vi "CAN总线测试.vi"() -> ()   [LabVIEW 2010]
uses:
  全局量/试验配置信息.vi
panel:
  in  "同步_2":i32
  in  "同步_1":i32
  out "CAN_R_4_4":u16
  out "CAN_R_4_3":u16
  out "CAN_R_4_2":u16
  out "CAN_R_4_1":u16
  out "CAN_R_3_4":u16
  out "CAN_R_3_3":u16
  out "CAN_R_3_2":u16
  out "CAN_R_3_1":u16
  out "CAN_R_2_4":u16
  out "CAN_R_2_3":u16
  out "CAN_R_2_2":u16
  out "CAN_R_2_1":u16
  out "CAN_R_1_4":u16
  out "CAN_R_1_3":u16
  out "CAN_R_1_2":u16
  out "CAN_R_1_1":u16
  out "结束?":bool
  out "light_4":bool
  out "light_3":bool
  out "light_2":bool
  out "light_1":bool
  out "测试结论":string
  in  "btn_关闭":bool
  in  "btn_开始测试":bool
  in  "CAN_4_4":u16
  in  "CAN_4_3":u16
  in  "CAN_4_2":u16
  in  "CAN_4_1":u16
  in  "单选_CAN_4":bool
  in  "CAN_3_4":u16
  in  "CAN_3_3":u16
  in  "CAN_3_2":u16
  in  "CAN_3_1":u16
  in  "单选_CAN_3":bool
  in  "CAN_2_4":u16
  in  "CAN_2_3":u16
  in  "CAN_2_2":u16
  in  "CAN_2_1":u16
  in  "单选_CAN_2":bool
  in  "CAN_1_4":u16
  in  "CAN_1_3":u16
  in  "CAN_1_2":u16
  in  "CAN_1_1":u16
  in  "单选_CAN_1":bool
  # "CAN以发送数据："
  # "CAN1"
  # "CAN2"
  # "CAN3"
  # "CAN4"
  # "CAN接收数据："
  # "CAN1"
  # "CAN2"
  # "CAN3"
  # "CAN4"
  # "测试结论："
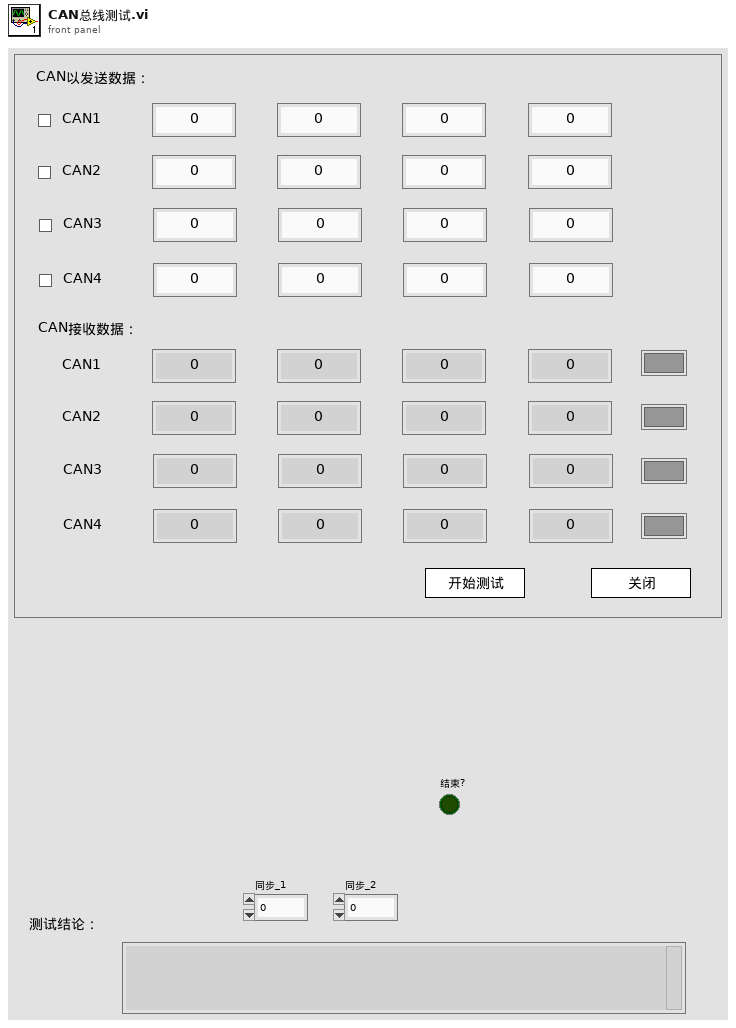
[diagram p1: front panel]
types:
  T1 = enum8{"Enabled", "Disabled", "Disabled and Grayed Out"}
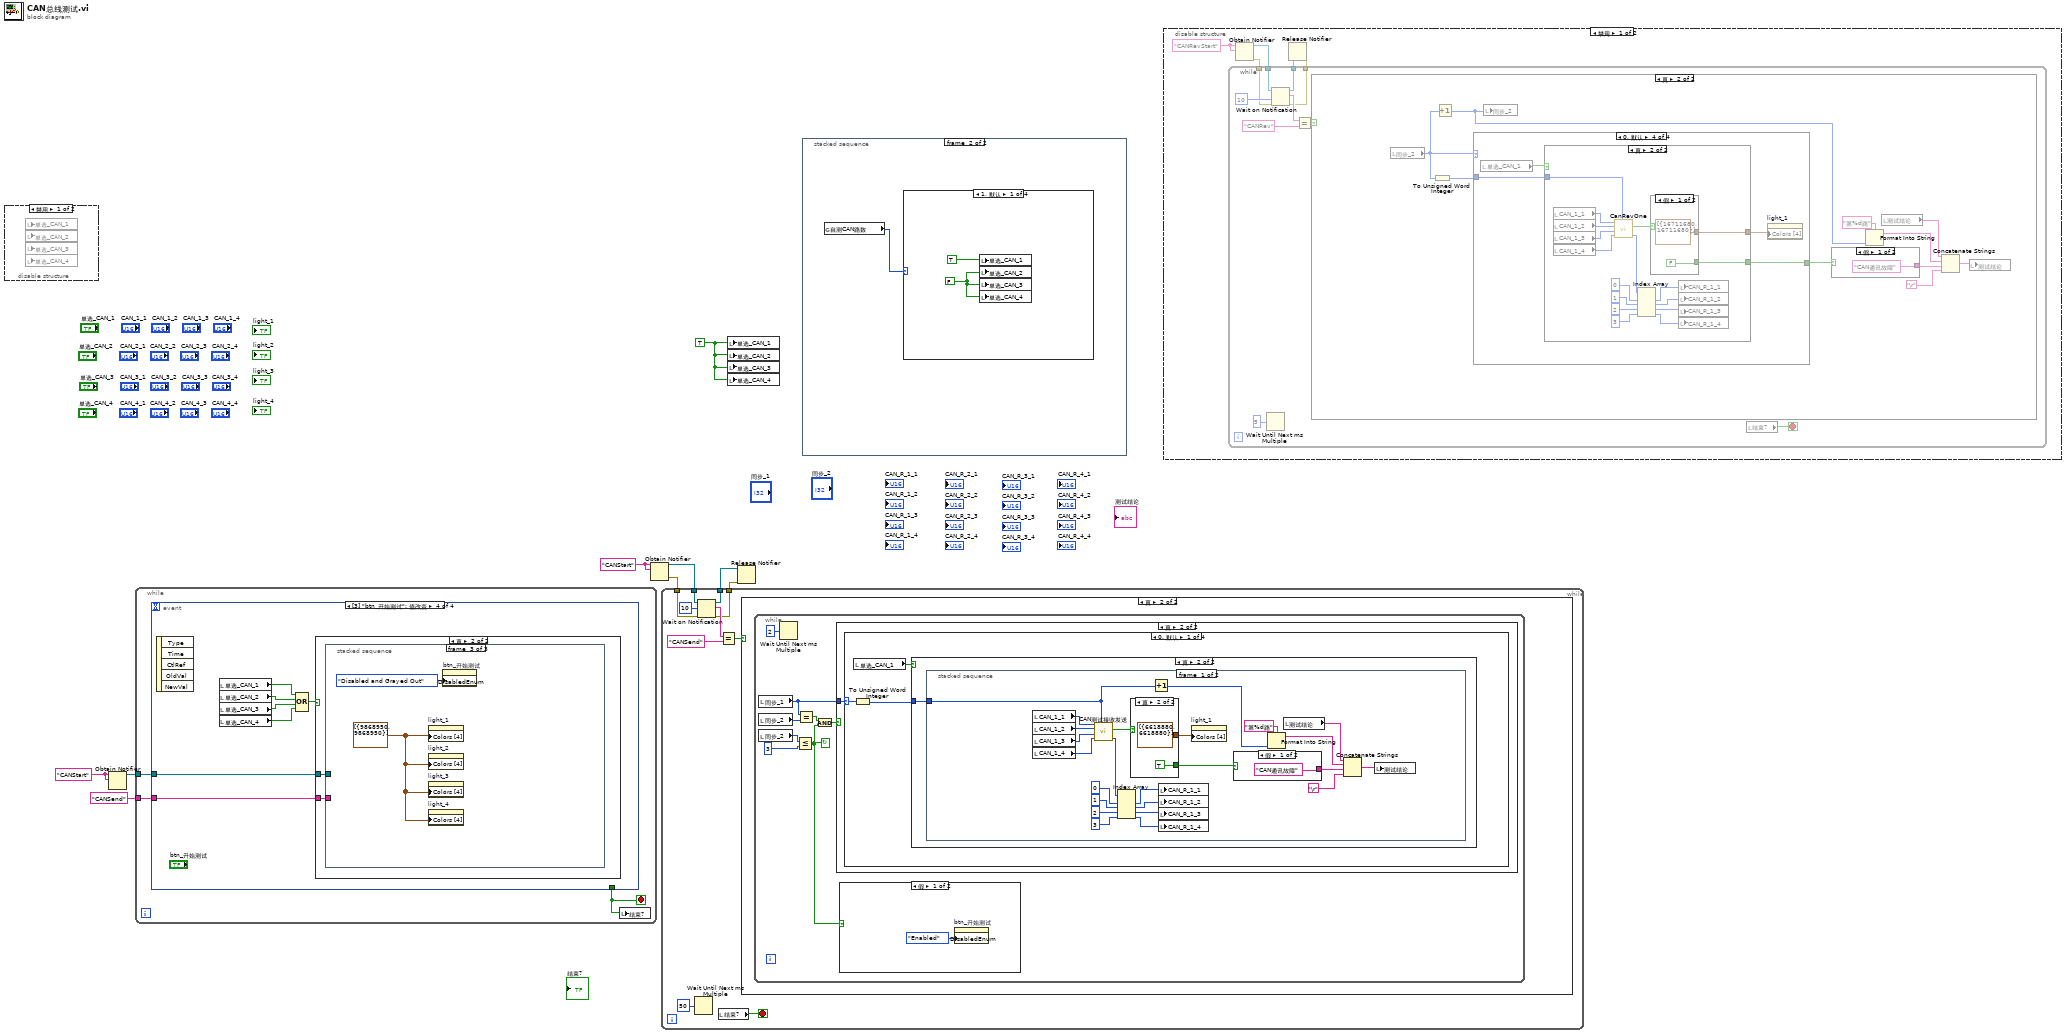
[diagram p0: block diagram]
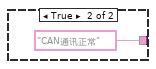
[diagram p3: hidden frame]
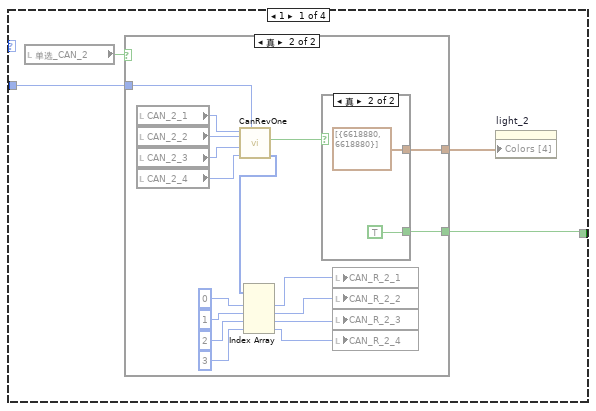
[diagram p4: hidden frame]
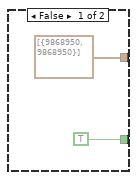
[diagram p5: hidden frame]
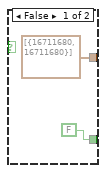
[diagram p6: hidden frame]
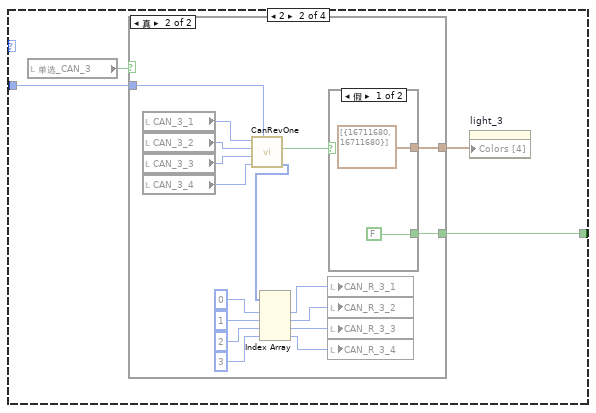
[diagram p7: hidden frame]
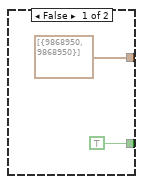
[diagram p8: hidden frame]
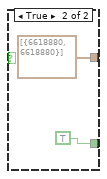
[diagram p9: hidden frame]
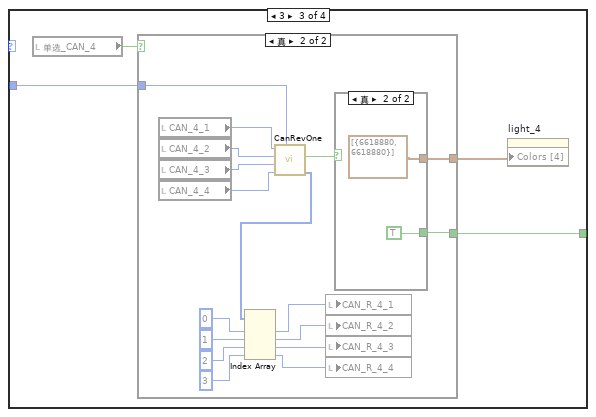
[diagram p10: hidden frame]
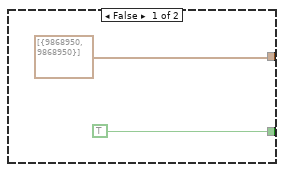
[diagram p11: hidden frame]
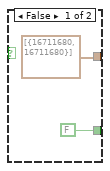
[diagram p12: hidden frame]
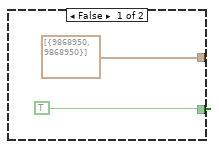
[diagram p13: hidden frame]
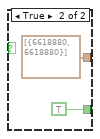
[diagram p14: hidden frame]
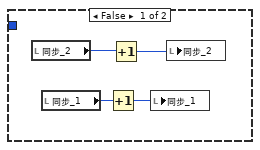
[diagram p19: hidden frame]
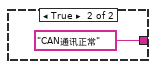
[diagram p20: hidden frame]
diagram:
  w1 = TRUE ("单选_CAN_1")
  w4 = "CANStart" ("名称（未命名）")
  w9 = "CANStart" ("名称（未命名）")
  n1 = disable-structure shown="禁用" {
    frame Disabled {
      n2 = local read "单选_CAN_1"() -> ()  [unwired: 1 in]
      n3 = local read "单选_CAN_2"() -> ()  [unwired: 1 in]
      n4 = local read "单选_CAN_3"() -> ()  [unwired: 1 in]
      n5 = local read "单选_CAN_4"() -> ()  [unwired: 1 in]
    }
    frame Enabled {
    }
  }
  n6 = Obtain Notifier(name (unnamed)=w4, notification data type=w4) -> (notifier out=w3:refnum<notifier>)  [unwired: 2 in, 2 out]
  n7 = while {
    tunnel: w3 -> [w11]
    tunnel: "CANSend" ("通知") -> [w10]
    stop <- w12 stop-if-true
    n8 = event shown="[3] \"btn_开始测试\": 值改变" {
      selector: _ -> [_ _ _ _]
      dyn-events: _ -> [_ _ _ _]
      timeout: _ -> [_ _ _ _]
      tunnel: [_ TRUE TRUE _] -> w12
      tunnel: w11 -> [_ _ _ w22]
      tunnel: w10 -> [_ _ _ w21]
      event Timeout {
        n9 = event-data() -> ()  [unwired: 1 in, 2 out]
      }
      event Panel Close {
        n10 = event-data() -> ()  [unwired: 1 in, 3 out]
        n11 = stacked-sequence {
          frame #0 {
            w14 = u16 0 ("CAN_R_1_1")
            w15 = 0 ("同步_2")
            w16 = cluster{u32, u32}[] [{9868950, 9868950}]
            n12 = local write "同步_2"(w15) -> ()
            n13 = local write "同步_1"(w15) -> ()
            n14 = property on="light_1" class="Bool (严格)"("Colors [4]"=w16) -> ()  [unwired: 2 in, 2 out]
            n15 = property on="light_2" class="Bool (严格)"("Colors [4]"=w16) -> ()  [unwired: 2 in, 2 out]
            n16 = property on="light_3" class="Bool (严格)"("Colors [4]"=w16) -> ()  [unwired: 2 in, 2 out]
            n17 = property on="light_4" class="Bool (严格)"("Colors [4]"=w16) -> ()  [unwired: 2 in, 2 out]
            n18 = local write "CAN_R_1_1"(w14) -> ()
            n19 = local write "CAN_R_1_2"(w14) -> ()
            n20 = local write "CAN_R_1_3"(w14) -> ()
            n21 = local write "CAN_R_1_4"(w14) -> ()
            n22 = local write "CAN_R_2_1"(w14) -> ()
            n23 = local write "CAN_R_2_2"(w14) -> ()
            n24 = local write "CAN_R_2_3"(w14) -> ()
            n25 = local write "CAN_R_2_4"(w14) -> ()
            n26 = local write "CAN_R_3_1"(w14) -> ()
            n27 = local write "CAN_R_3_2"(w14) -> ()
            n28 = local write "CAN_R_3_3"(w14) -> ()
            n29 = local write "CAN_R_3_4"(w14) -> ()
            n30 = local write "CAN_R_4_1"(w14) -> ()
            n31 = local write "CAN_R_4_2"(w14) -> ()
            n32 = local write "CAN_R_4_3"(w14) -> ()
            n33 = local write "CAN_R_4_4"(w14) -> ()
          }
        }
      }
      event "btn_关闭": Value Change {
        n34 = event-data() -> ()  [unwired: 1 in, 5 out]
        n35 = stacked-sequence {
          frame #0 {
            w18 = u16 0 ("CAN_R_1_1")
            w19 = 0 ("同步_2")
            w20 = cluster{u32, u32}[] [{9868950, 9868950}]
            n36 = local write "同步_2"(w19) -> ()
            n37 = local write "同步_1"(w19) -> ()
            n38 = property on="light_1" class="Bool (严格)"("Colors [4]"=w20) -> ()  [unwired: 2 in, 2 out]
            n39 = property on="light_2" class="Bool (严格)"("Colors [4]"=w20) -> ()  [unwired: 2 in, 2 out]
            n40 = property on="light_3" class="Bool (严格)"("Colors [4]"=w20) -> ()  [unwired: 2 in, 2 out]
            n41 = property on="light_4" class="Bool (严格)"("Colors [4]"=w20) -> ()  [unwired: 2 in, 2 out]
            n42 = local write "CAN_R_1_1"(w18) -> ()
            n43 = local write "CAN_R_1_2"(w18) -> ()
            n44 = local write "CAN_R_1_3"(w18) -> ()
            n45 = local write "CAN_R_1_4"(w18) -> ()
            n46 = local write "CAN_R_2_1"(w18) -> ()
            n47 = local write "CAN_R_2_2"(w18) -> ()
            n48 = local write "CAN_R_2_3"(w18) -> ()
            n49 = local write "CAN_R_2_4"(w18) -> ()
            n50 = local write "CAN_R_3_1"(w18) -> ()
            n51 = local write "CAN_R_3_2"(w18) -> ()
            n52 = local write "CAN_R_3_3"(w18) -> ()
            n53 = local write "CAN_R_3_4"(w18) -> ()
            n54 = local write "CAN_R_4_1"(w18) -> ()
            n55 = local write "CAN_R_4_2"(w18) -> ()
            n56 = local write "CAN_R_4_3"(w18) -> ()
            n57 = local write "CAN_R_4_4"(w18) -> ()
          }
        }
      }
      event "btn_开始测试": Value Change {
        n58 = event-data() -> ()  [unwired: 1 in, 5 out]
        n59 = local read "单选_CAN_1"() -> (w27:bool)
        n60 = local read "单选_CAN_2"() -> (w26:bool)
        n61 = local read "单选_CAN_3"() -> (w25:bool)
        n62 = local read "单选_CAN_4"() -> (w24:bool)
        n63 = Compound Arithmetic op=OR(w27, w26, w25, w24) -> (w23:bool)
        n64 = case shown="真" w23 {
          tunnel: w22 -> [_ w29]
          tunnel: w21 -> [_ w28]
          frame False {
            n65 = call "显示对话框信息"() -> ()  [unwired: 10 in, 2 out]
          }
          frame True {
            n66 = stacked-sequence {
              tunnel: w29 -> [_ w34 _]
              tunnel: w28 -> [_ w33 _]
              frame #0 {
                w30 = u16 0 ("CAN_R_1_1")
                w31 = 0 ("同步_2")
                n67 = local write "同步_2"(w31) -> ()
                n68 = local write "同步_1"(w31) -> ()
                n69 = local write "测试结论"("") -> ()
                n70 = local write "CAN_R_1_1"(w30) -> ()
                n71 = local write "CAN_R_1_2"(w30) -> ()
                n72 = local write "CAN_R_1_3"(w30) -> ()
                n73 = local write "CAN_R_1_4"(w30) -> ()
                n74 = local write "CAN_R_2_1"(w30) -> ()
                n75 = local write "CAN_R_2_2"(w30) -> ()
                n76 = local write "CAN_R_2_3"(w30) -> ()
                n77 = local write "CAN_R_2_4"(w30) -> ()
                n78 = local write "CAN_R_3_1"(w30) -> ()
                n79 = local write "CAN_R_3_2"(w30) -> ()
                n80 = local write "CAN_R_3_3"(w30) -> ()
                n81 = local write "CAN_R_3_4"(w30) -> ()
                n82 = local write "CAN_R_4_1"(w30) -> ()
                n83 = local write "CAN_R_4_2"(w30) -> ()
                n84 = local write "CAN_R_4_3"(w30) -> ()
                n85 = local write "CAN_R_4_4"(w30) -> ()
              }
              frame #1 {
                n86 = Send Notification(notification=w33, notifier=w34) -> ()  [unwired: 1 in, 2 out]
              }
              frame #2 {
                w35 = cluster{u32, u32}[] [{9868950, 9868950}]
                n87 = property on="light_1" class="Bool (严格)"("Colors [4]"=w35) -> ()  [unwired: 2 in, 2 out]
                n88 = property on="light_2" class="Bool (严格)"("Colors [4]"=w35) -> ()  [unwired: 2 in, 2 out]
                n89 = property on="light_3" class="Bool (严格)"("Colors [4]"=w35) -> ()  [unwired: 2 in, 2 out]
                n90 = property on="light_4" class="Bool (严格)"("Colors [4]"=w35) -> ()  [unwired: 2 in, 2 out]
                n91 = property on="btn_开始测试" class="Bool"("DisabledEnum"=T1."Disabled and Grayed Out" ("禁用")) -> ()  [unwired: 2 in, 2 out]
              }
            }
          }
        }
      }
    }
    n92 = local write "结束?"(w12) -> ()
  }
  n93 = Obtain Notifier(name (unnamed)=w9, notification data type=w9) -> (notifier out=w7:refnum<notifier>, error out=w8:errorcluster)  [unwired: 2 in, 1 out]
  n94 = while {
    tunnel: w8 -> [w40]
    tunnel: w7 -> [w39]
    tunnel: [w38] -> w6
    tunnel: [w37] -> w5
    stop <- w45 stop-if-true
    n95 = Wait Until Next ms Multiple(millisecond multiple=u32 50 ("毫秒倍数")) -> ()  [unwired: 1 out]
    n96 = Wait on Notification(notifier=w39, timeout in ms (-1)=10 ("超时毫秒(-1)"), error in (no error)=w40) -> (notifier out=w38:refnum<notifier>, notification=w42:string, error out=w37:errorcluster)  [unwired: 1 in, 1 out]
    n97 = local read "结束?"() -> (w45:bool)
    n98 = Equal?(x=w42, y="CANSend" ("通知")) -> (x = y?=w41:bool)
    n99 = case shown="真" w41 {
      frame False {
      }
      frame True {
        n100 = while {
          stop <- w47 continue-if-true
          n101 = local read "同步_1"() -> (w54:i32)
          n102 = local read "同步_2"() -> (w50:i32)
          n103 = local read "同步_2"() -> (w52:i32)
          n104 = Wait Until Next ms Multiple(millisecond multiple=u32 2 ("毫秒倍数")) -> ()  [unwired: 1 out]
          n105 = Less Or Equal?(x=w52, y=3) -> (x <= y?=w47:bool)
          n106 = Equal?(x=w54, y=w50) -> (x = y?=w48:bool)
          n107 = And(x=w48, y=w47) -> (x .and. y?=w49:bool)
          n108 = case shown="真" w49 {
            tunnel: w54 -> [_ w56]
            frame False {
            }
            frame True {
              n109 = case shown="0, 默认" w56 {
                selector: w56 -> [w57 w101 w143 w185]
                frame 0, Default {
                  n110 = local read "单选_CAN_1"() -> (w59:bool)
                  n111 = To Unsigned Word Integer(number=w57) -> (unsigned 16bit integer=w58:u16)
                  n112 = case shown="真" w59 {
                    tunnel: w58 -> [_ w64]
                    frame False {
                      n113 = local read "同步_2"() -> (w62:i32)
                      n114 = local read "同步_1"() -> (w60:i32)
                      n115 = Increment(x=w60) -> (x+1=w61:i32)
                      n116 = Increment(x=w62) -> (x+1=w63:i32)
                      n117 = local write "同步_1"(w61) -> ()
                      n118 = local write "同步_2"(w63) -> ()
                    }
                    frame True {
                      n119 = stacked-sequence {
                        tunnel: w64 -> [w65 _]
                        frame #0 {
                          n120 = local read "CAN_1_1"() -> (w75:u16)
                          n121 = local read "CAN_1_2"() -> (w76:u16)
                          n122 = local read "CAN_1_3"() -> (w77:u16)
                          n123 = local read "CAN_1_4"() -> (w78:u16)
                          n124 = call "CAN测试接收发送.vi"("Order"=w65, "data_4"=w78, "data_3"=w77, "data_2"=w76, "data_1"=w75) -> ("接收数据"=w80:u16[], "成功？"=w79:bool)  [unwired: 5 in]
                          n125 = Index Array(array=w80, index #1=0 ("索引"), index #2=1 ("索引"), index #3=2 ("索引"), index #4=3 ("索引")) -> (element #1=w85:u16, element #2=w86:u16, element #3=w87:u16, element #4=w88:u16)
                          n126 = case shown="真" w79 {
                            tunnel: [cluster{u32, u32}[] [{16711680, 16711680}] cluster{u32, u32}[] [{6618880, 6618880}]] -> w74
                            tunnel: [FALSE TRUE] -> w66
                            frame False {
                            }
                            frame True {
                            }
                          }
                          n127 = Increment(x=w65) -> (x+1=w67:u16)
                          n128 = local write "CAN_R_1_1"(w85) -> ()
                          n129 = local write "CAN_R_1_2"(w86) -> ()
                          n130 = local write "CAN_R_1_3"(w87) -> ()
                          n131 = local write "CAN_R_1_4"(w88) -> ()
                          n132 = property on="light_1" class="Bool (严格)"("Colors [4]"=w74) -> ()  [unwired: 2 in, 2 out]
                          n133 = case shown="假" w66 {
                            tunnel: ["CAN通讯故障" "CAN通讯正常"] -> w70
                            frame False {
                            }
                            frame True {
                            }
                          }
                          n134 = Format Into String(format string="第%d路", w67) -> (resulting string=w71:string)  [unwired: 2 in, 1 out]
                          n135 = local read "测试结论"() -> (w72:string)
                          n136 = Concatenate Strings(w72, w71, w70, "\r") -> (w68:string)
                          n137 = local write "测试结论"(w68) -> ()
                        }
                        frame #1 {
                          n138 = local read "同步_1"() -> (w97:i32)
                          n139 = local read "同步_2"() -> (w95:i32)
                          n140 = Increment(x=w97) -> (x+1=w98:i32)
                          n141 = Increment(x=w95) -> (x+1=w96:i32)
                          n142 = local write "同步_2"(w96) -> ()
                          n143 = local write "同步_1"(w98) -> ()
                        }
                      }
                    }
                  }
                }
                frame 1 {
                  n144 = local read "单选_CAN_2"() -> (w100:bool)
                  n145 = To Unsigned Word Integer(number=w101) -> (unsigned 16bit integer=w99:u16)
                  n146 = case shown="真" w100 {
                    tunnel: w99 -> [_ w106]
                    frame False {
                      n147 = local read "同步_2"() -> (w104:i32)
                      n148 = local read "同步_1"() -> (w102:i32)
                      n149 = Increment(x=w102) -> (x+1=w103:i32)
                      n150 = Increment(x=w104) -> (x+1=w105:i32)
                      n151 = local write "同步_1"(w103) -> ()
                      n152 = local write "同步_2"(w105) -> ()
                    }
                    frame True {
                      n153 = stacked-sequence {
                        tunnel: w106 -> [w130 _]
                        frame #0 {
                          n154 = local read "CAN_2_1"() -> (w116:u16)
                          n155 = local read "CAN_2_2"() -> (w117:u16)
                          n156 = local read "CAN_2_3"() -> (w118:u16)
                          n157 = local read "CAN_2_4"() -> (w119:u16)
                          n158 = call "CAN测试接收发送.vi"("Order"=w130, "data_4"=w119, "data_3"=w118, "data_2"=w117, "data_1"=w116) -> ("接收数据"=w125:u16[], "成功？"=w120:bool)  [unwired: 5 in]
                          n159 = Index Array(array=w125, index #1=0 ("索引"), index #2=1 ("索引"), index #3=2 ("索引"), index #4=3 ("索引")) -> (element #1=w126:u16, element #2=w127:u16, element #3=w128:u16, element #4=w129:u16)
                          n160 = case shown="真" w120 {
                            tunnel: [cluster{u32, u32}[] [{16711680, 16711680}] cluster{u32, u32}[] [{6618880, 6618880}]] -> w115
                            tunnel: [FALSE TRUE] -> w108
                            frame False {
                            }
                            frame True {
                            }
                          }
                          n161 = local write "CAN_R_2_1"(w126) -> ()
                          n162 = local write "CAN_R_2_2"(w127) -> ()
                          n163 = local write "CAN_R_2_3"(w128) -> ()
                          n164 = local write "CAN_R_2_4"(w129) -> ()
                          n165 = Increment(x=w130) -> (x+1=w107:u16)
                          n166 = property on="light_2" class="Bool (严格)"("Colors [4]"=w115) -> ()  [unwired: 2 in, 2 out]
                          n167 = case shown="假" w108 {
                            tunnel: ["CAN通讯故障" "CAN通讯正常"] -> w112
                            frame False {
                            }
                            frame True {
                            }
                          }
                          n168 = Format Into String(format string="第%d路", w107) -> (resulting string=w111:string)  [unwired: 2 in, 1 out]
                          n169 = local read "测试结论"() -> (w110:string)
                          n170 = Concatenate Strings(w110, w111, w112, "\r") -> (w114:string)
                          n171 = local write "测试结论"(w114) -> ()
                        }
                        frame #1 {
                          n172 = local read "同步_1"() -> (w139:i32)
                          n173 = local read "同步_2"() -> (w138:i32)
                          n174 = Increment(x=w139) -> (x+1=w140:i32)
                          n175 = Increment(x=w138) -> (x+1=w137:i32)
                          n176 = local write "同步_2"(w137) -> ()
                          n177 = local write "同步_1"(w140) -> ()
                        }
                      }
                    }
                  }
                }
                frame 2 {
                  n178 = local read "单选_CAN_3"() -> (w142:bool)
                  n179 = To Unsigned Word Integer(number=w143) -> (unsigned 16bit integer=w141:u16)
                  n180 = case shown="真" w142 {
                    tunnel: w141 -> [_ w148]
                    frame False {
                      n181 = local read "同步_1"() -> (w144:i32)
                      n182 = local read "同步_2"() -> (w146:i32)
                      n183 = Increment(x=w144) -> (x+1=w145:i32)
                      n184 = Increment(x=w146) -> (x+1=w147:i32)
                      n185 = local write "同步_1"(w145) -> ()
                      n186 = local write "同步_2"(w147) -> ()
                    }
                    frame True {
                      n187 = stacked-sequence {
                        tunnel: w148 -> [w172 _]
                        frame #0 {
                          n188 = local read "CAN_3_1"() -> (w158:u16)
                          n189 = local read "CAN_3_2"() -> (w159:u16)
                          n190 = local read "CAN_3_3"() -> (w160:u16)
                          n191 = local read "CAN_3_4"() -> (w161:u16)
                          n192 = call "CAN测试接收发送.vi"("Order"=w172, "data_4"=w161, "data_3"=w160, "data_2"=w159, "data_1"=w158) -> ("接收数据"=w167:u16[], "成功？"=w162:bool)  [unwired: 5 in]
                          n193 = Index Array(array=w167, index #1=0 ("索引"), index #2=1 ("索引"), index #3=2 ("索引"), index #4=3 ("索引")) -> (element #1=w168:u16, element #2=w169:u16, element #3=w170:u16, element #4=w171:u16)
                          n194 = local write "CAN_R_3_1"(w168) -> ()
                          n195 = local write "CAN_R_3_2"(w169) -> ()
                          n196 = local write "CAN_R_3_3"(w170) -> ()
                          n197 = local write "CAN_R_3_4"(w171) -> ()
                          n198 = case shown="真" w162 {
                            tunnel: [cluster{u32, u32}[] [{16711680, 16711680}] cluster{u32, u32}[] [{6618880, 6618880}]] -> w157
                            tunnel: [FALSE TRUE] -> w149
                            frame False {
                            }
                            frame True {
                            }
                          }
                          n199 = Increment(x=w172) -> (x+1=w150:u16)
                          n200 = property on="light_3" class="Bool (严格)"("Colors [4]"=w157) -> ()  [unwired: 2 in, 2 out]
                          n201 = case shown="假" w149 {
                            tunnel: ["CAN通讯故障" "CAN通讯正常"] -> w154
                            frame False {
                            }
                            frame True {
                            }
                          }
                          n202 = Format Into String(format string="第%d路", w150) -> (resulting string=w153:string)  [unwired: 2 in, 1 out]
                          n203 = local read "测试结论"() -> (w152:string)
                          n204 = Concatenate Strings(w152, w153, w154, "\r") -> (w156:string)
                          n205 = local write "测试结论"(w156) -> ()
                        }
                        frame #1 {
                          n206 = local read "同步_1"() -> (w181:i32)
                          n207 = local read "同步_2"() -> (w179:i32)
                          n208 = Increment(x=w181) -> (x+1=w182:i32)
                          n209 = Increment(x=w179) -> (x+1=w180:i32)
                          n210 = local write "同步_1"(w182) -> ()
                          n211 = local write "同步_2"(w180) -> ()
                        }
                      }
                    }
                  }
                }
                frame 3 {
                  n212 = local read "单选_CAN_4"() -> (w184:bool)
                  n213 = To Unsigned Word Integer(number=w185) -> (unsigned 16bit integer=w183:u16)
                  n214 = case shown="真" w184 {
                    tunnel: w183 -> [_ w190]
                    frame False {
                      n215 = local read "同步_2"() -> (w188:i32)
                      n216 = local read "同步_1"() -> (w187:i32)
                      n217 = Increment(x=w188) -> (x+1=w189:i32)
                      n218 = Increment(x=w187) -> (x+1=w186:i32)
                      n219 = local write "同步_1"(w186) -> ()
                      n220 = local write "同步_2"(w189) -> ()
                    }
                    frame True {
                      n221 = stacked-sequence {
                        tunnel: w190 -> [w214 _]
                        frame #0 {
                          n222 = local read "CAN_4_1"() -> (w213:u16)
                          n223 = local read "CAN_4_2"() -> (w212:u16)
                          n224 = local read "CAN_4_3"() -> (w211:u16)
                          n225 = local read "CAN_4_4"() -> (w210:u16)
                          n226 = call "CAN测试接收发送.vi"("Order"=w214, "data_4"=w210, "data_3"=w211, "data_2"=w212, "data_1"=w213) -> ("接收数据"=w204:u16[], "成功？"=w209:bool)  [unwired: 5 in]
                          n227 = Index Array(array=w204, index #1=0 ("索引"), index #2=1 ("索引"), index #3=2 ("索引"), index #4=3 ("索引")) -> (element #1=w203:u16, element #2=w202:u16, element #3=w201:u16, element #4=w200:u16)
                          n228 = local write "CAN_R_4_1"(w203) -> ()
                          n229 = local write "CAN_R_4_2"(w202) -> ()
                          n230 = local write "CAN_R_4_3"(w201) -> ()
                          n231 = local write "CAN_R_4_4"(w200) -> ()
                          n232 = case shown="真" w209 {
                            tunnel: [cluster{u32, u32}[] [{16711680, 16711680}] cluster{u32, u32}[] [{6618880, 6618880}]] -> w199
                            tunnel: [FALSE TRUE] -> w191
                            frame False {
                            }
                            frame True {
                            }
                          }
                          n233 = Increment(x=w214) -> (x+1=w192:u16)
                          n234 = property on="light_4" class="Bool (严格)"("Colors [4]"=w199) -> ()  [unwired: 2 in, 2 out]
                          n235 = case shown="假" w191 {
                            tunnel: ["CAN通讯故障" "CAN通讯正常"] -> w196
                            frame False {
                            }
                            frame True {
                            }
                          }
                          n236 = Format Into String(format string="第%d路", w192) -> (resulting string=w195:string)  [unwired: 2 in, 1 out]
                          n237 = local read "测试结论"() -> (w194:string)
                          n238 = Concatenate Strings(w194, w195, w196, "\r") -> (w198:string)
                          n239 = local write "测试结论"(w198) -> ()
                        }
                        frame #1 {
                          n240 = local read "同步_1"() -> (w224:i32)
                          n241 = local read "同步_2"() -> (w221:i32)
                          n242 = Increment(x=w224) -> (x+1=w223:i32)
                          n243 = Increment(x=w221) -> (x+1=w222:i32)
                          n244 = local write "同步_2"(w222) -> ()
                          n245 = local write "同步_1"(w223) -> ()
                        }
                      }
                    }
                  }
                }
              }
            }
          }
          n246 = case shown="假" w47 {
            frame False {
              n247 = property on="btn_开始测试" class="Bool"("DisabledEnum"=T1."Enabled" ("禁用")) -> ()  [unwired: 2 in, 2 out]
            }
            frame True {
            }
          }
        }
      }
    }
  }
  n248 = local write "单选_CAN_1"(w1) -> ()
  n249 = local write "单选_CAN_2"(w1) -> ()
  n250 = local write "单选_CAN_3"(w1) -> ()
  n251 = local write "单选_CAN_4"(w1) -> ()
  n252 = Release Notifier(notifier=w6, error in (no error)=w5) -> ()  [unwired: 1 in, 3 out]
  n253 = stacked-sequence {
    frame #0 {
      w226 = TRUE ("单选_CAN_1")
      w227 = 0 ("同步_2")
      w229 = cluster{u32, u32}[] [{9868950, 9868950}]
      n254 = local write "结束?"(FALSE ("结束?")) -> ()
      n255 = local write "同步_2"(w227) -> ()
      n256 = local write "同步_1"(w227) -> ()
      n257 = property on="light_1" class="Bool (严格)"("Colors [4]"=w229) -> ()  [unwired: 2 in, 2 out]
      n258 = property on="light_2" class="Bool (严格)"("Colors [4]"=w229) -> ()  [unwired: 2 in, 2 out]
      n259 = property on="light_3" class="Bool (严格)"("Colors [4]"=w229) -> ()  [unwired: 2 in, 2 out]
      n260 = property on="light_4" class="Bool (严格)"("Colors [4]"=w229) -> ()  [unwired: 2 in, 2 out]
      n261 = local write "单选_CAN_1"(w226) -> ()
      n262 = local write "单选_CAN_2"(w226) -> ()
      n263 = local write "单选_CAN_3"(w226) -> ()
      n264 = local write "单选_CAN_4"(w226) -> ()
      n265 = for {
        N: 16 -> [_]
        i -> [w231]
        n266 = Multiply(x=3 ("CAN_R_1_1"), y=w231) -> (x*y=w230:i32)
        n267 = case shown="15" w231 {
          tunnel: w230 -> [w233 w234 w235 w236 w237 w238 w239 w240 w241 w242 w243 w244 w245 w246 w247 w248]
          frame 0, Default {
            n268 = local write "CAN_1_1"(w233) -> ()
          }
          frame 1 {
            n269 = local write "CAN_1_2"(w234) -> ()
          }
          frame 2 {
            n270 = local write "CAN_1_3"(w235) -> ()
          }
          frame 3 {
            n271 = local write "CAN_1_4"(w236) -> ()
          }
          frame 4 {
            n272 = local write "CAN_2_1"(w237) -> ()
          }
          frame 5 {
            n273 = local write "CAN_2_2"(w238) -> ()
          }
          frame 6 {
            n274 = local write "CAN_2_3"(w239) -> ()
          }
          frame 7 {
            n275 = local write "CAN_2_4"(w240) -> ()
          }
          frame 8 {
            n276 = local write "CAN_3_1"(w241) -> ()
          }
          frame 9 {
            n277 = local write "CAN_3_2"(w242) -> ()
          }
          frame 10 {
            n278 = local write "CAN_3_3"(w243) -> ()
          }
          frame 11 {
            n279 = local write "CAN_3_4"(w244) -> ()
          }
          frame 12 {
            n280 = local write "CAN_4_1"(w245) -> ()
          }
          frame 13 {
            n281 = local write "CAN_4_2"(w246) -> ()
          }
          frame 14 {
            n282 = local write "CAN_4_3"(w247) -> ()
          }
          frame 15 {
            n283 = local write "CAN_4_4"(w248) -> ()
          }
        }
      }
    }
    frame #1 {
      n284 = global read "试验配置信息.vi" "自测CAN路数"() -> (w249:i32)
      n285 = case shown="1, 默认" w249 {
        frame 1, Default {
          w250 = FALSE
          n286 = local write "单选_CAN_1"(TRUE ("单选_CAN_1")) -> ()
          n287 = local write "单选_CAN_2"(w250) -> ()
          n288 = local write "单选_CAN_3"(w250) -> ()
          n289 = local write "单选_CAN_4"(w250) -> ()
        }
        frame 2 {
          w253 = FALSE
          w252 = TRUE ("单选_CAN_1")
          n290 = local write "单选_CAN_1"(w252) -> ()
          n291 = local write "单选_CAN_2"(w252) -> ()
          n292 = local write "单选_CAN_3"(w253) -> ()
          n293 = local write "单选_CAN_4"(w253) -> ()
        }
        frame 3 {
          w254 = TRUE ("单选_CAN_1")
          n294 = local write "单选_CAN_1"(w254) -> ()
          n295 = local write "单选_CAN_2"(w254) -> ()
          n296 = local write "单选_CAN_3"(w254) -> ()
          n297 = local write "单选_CAN_4"(FALSE) -> ()
        }
        frame 4 {
          w256 = TRUE ("单选_CAN_1")
          n298 = local write "单选_CAN_1"(w256) -> ()
          n299 = local write "单选_CAN_2"(w256) -> ()
          n300 = local write "单选_CAN_3"(w256) -> ()
          n301 = local write "单选_CAN_4"(w256) -> ()
        }
      }
    }
  }
  n302 = disable-structure shown="禁用" {
    frame Disabled {
      w261 = "CANRevStart" ("名称（未命名）")
      n303 = Obtain Notifier(name (unnamed)=w261, notification data type=w261) -> (notifier out=w259:refnum<notifier>, error out=w260:errorcluster)  [unwired: 2 in, 1 out]
      n304 = while {
        tunnel: w260 -> [w266]
        tunnel: w259 -> [w265]
        tunnel: [w264] -> w258
        tunnel: [w263] -> w257
        stop <- w271 stop-if-true
        n305 = Wait Until Next ms Multiple(millisecond multiple=u32 5 ("毫秒倍数")) -> ()  [unwired: 1 out]
        n306 = Wait on Notification(notifier=w265, timeout in ms (-1)=10 ("超时毫秒(-1)"), error in (no error)=w266) -> (notifier out=w264:refnum<notifier>, notification=w268:string, error out=w263:errorcluster)  [unwired: 1 in, 1 out]
        n307 = Equal?(x=w268, y="CANRev" ("通知")) -> (x = y?=w262:bool)
        n308 = case shown="真" w262 {
          frame False {
          }
          frame True {
            n309 = local read "同步_2"() -> (w281:i32)
            n310 = To Unsigned Word Integer(number=w281) -> (unsigned 16bit integer=w280:u16)
            n311 = Increment(x=w281) -> (x+1=w273:i32)
            n312 = case shown="0, 默认" w281 {
              tunnel: w280 -> [w286 w313 w340 w367]
              tunnel: [w284 w311 w338 w365] -> w274
              frame 1 {
                n313 = local read "单选_CAN_2"() -> (w287:bool)
                n314 = case shown="真" w287 {
                  tunnel: w286 -> [_ w306]
                  tunnel: [TRUE w300] -> w284
                  tunnel: [cluster{u32, u32}[] [{9868950, 9868950}] w294] -> w285
                  frame False {
                  }
                  frame True {
                    n315 = local read "CAN_2_1"() -> (w305:u16)
                    n316 = local read "CAN_2_2"() -> (w304:u16)
                    n317 = local read "CAN_2_3"() -> (w303:u16)
                    n318 = local read "CAN_2_4"() -> (w302:u16)
                    n319 = call "CanRevOne.vi"("CANPort"=w306, "data_4"=w302, "data_3"=w303, "data_2"=w304, "data_1"=w305) -> ("接收数据"=w295:u16[], "成功？"=w301:bool)  [unwired: 5 in]
                    n320 = Index Array(array=w295, index #1=0 ("索引"), index #2=1 ("索引"), index #3=2 ("索引"), index #4=3 ("索引")) -> (element #1=w293:u16, element #2=w292:u16, element #3=w291:u16, element #4=w290:u16)
                    n321 = case shown="真" w301 {
                      tunnel: [cluster{u32, u32}[] [{16711680, 16711680}] cluster{u32, u32}[] [{6618880, 6618880}]] -> w294
                      tunnel: [FALSE TRUE] -> w300
                      frame False {
                      }
                      frame True {
                      }
                    }
                    n322 = local write "CAN_R_2_1"(w293) -> ()
                    n323 = local write "CAN_R_2_2"(w292) -> ()
                    n324 = local write "CAN_R_2_3"(w291) -> ()
                    n325 = local write "CAN_R_2_4"(w290) -> ()
                  }
                }
                n326 = property on="light_2" class="Bool (严格)"("Colors [4]"=w285) -> ()  [unwired: 2 in, 2 out]
              }
              frame 2 {
                n327 = local read "单选_CAN_3"() -> (w314:bool)
                n328 = case shown="真" w314 {
                  tunnel: w313 -> [_ w333]
                  tunnel: [TRUE w327] -> w311
                  tunnel: [cluster{u32, u32}[] [{9868950, 9868950}] w321] -> w312
                  frame False {
                  }
                  frame True {
                    n329 = local read "CAN_3_1"() -> (w332:u16)
                    n330 = local read "CAN_3_2"() -> (w331:u16)
                    n331 = local read "CAN_3_3"() -> (w330:u16)
                    n332 = local read "CAN_3_4"() -> (w329:u16)
                    n333 = call "CanRevOne.vi"("CANPort"=w333, "data_4"=w329, "data_3"=w330, "data_2"=w331, "data_1"=w332) -> ("接收数据"=w322:u16[], "成功？"=w328:bool)  [unwired: 5 in]
                    n334 = Index Array(array=w322, index #1=0 ("索引"), index #2=1 ("索引"), index #3=2 ("索引"), index #4=3 ("索引")) -> (element #1=w320:u16, element #2=w319:u16, element #3=w318:u16, element #4=w317:u16)
                    n335 = local write "CAN_R_3_1"(w320) -> ()
                    n336 = local write "CAN_R_3_2"(w319) -> ()
                    n337 = local write "CAN_R_3_3"(w318) -> ()
                    n338 = local write "CAN_R_3_4"(w317) -> ()
                    n339 = case shown="假" w328 {
                      tunnel: [cluster{u32, u32}[] [{16711680, 16711680}] cluster{u32, u32}[] [{6618880, 6618880}]] -> w321
                      tunnel: [FALSE TRUE] -> w327
                      frame False {
                      }
                      frame True {
                      }
                    }
                  }
                }
                n340 = property on="light_3" class="Bool (严格)"("Colors [4]"=w312) -> ()  [unwired: 2 in, 2 out]
              }
              frame 3 {
                n341 = local read "单选_CAN_4"() -> (w341:bool)
                n342 = case shown="真" w341 {
                  tunnel: w340 -> [_ w360]
                  tunnel: [TRUE w354] -> w338
                  tunnel: [cluster{u32, u32}[] [{9868950, 9868950}] w348] -> w339
                  frame False {
                  }
                  frame True {
                    n343 = local read "CAN_4_1"() -> (w359:u16)
                    n344 = local read "CAN_4_2"() -> (w358:u16)
                    n345 = local read "CAN_4_3"() -> (w357:u16)
                    n346 = local read "CAN_4_4"() -> (w356:u16)
                    n347 = call "CanRevOne.vi"("CANPort"=w360, "data_4"=w356, "data_3"=w357, "data_2"=w358, "data_1"=w359) -> ("接收数据"=w349:u16[], "成功？"=w355:bool)  [unwired: 5 in]
                    n348 = Index Array(array=w349, index #1=0 ("索引"), index #2=1 ("索引"), index #3=2 ("索引"), index #4=3 ("索引")) -> (element #1=w347:u16, element #2=w346:u16, element #3=w345:u16, element #4=w344:u16)
                    n349 = local write "CAN_R_4_1"(w347) -> ()
                    n350 = local write "CAN_R_4_2"(w346) -> ()
                    n351 = local write "CAN_R_4_3"(w345) -> ()
                    n352 = local write "CAN_R_4_4"(w344) -> ()
                    n353 = case shown="真" w355 {
                      tunnel: [cluster{u32, u32}[] [{16711680, 16711680}] cluster{u32, u32}[] [{6618880, 6618880}]] -> w348
                      tunnel: [FALSE TRUE] -> w354
                      frame False {
                      }
                      frame True {
                      }
                    }
                  }
                }
                n354 = property on="light_4" class="Bool (严格)"("Colors [4]"=w339) -> ()  [unwired: 2 in, 2 out]
              }
              frame 0, Default {
                n355 = local read "单选_CAN_1"() -> (w368:bool)
                n356 = case shown="真" w368 {
                  tunnel: w367 -> [_ w387]
                  tunnel: [TRUE w381] -> w365
                  tunnel: [cluster{u32, u32}[] [{9868950, 9868950}] w375] -> w366
                  frame False {
                  }
                  frame True {
                    n357 = local read "CAN_1_1"() -> (w386:u16)
                    n358 = local read "CAN_1_2"() -> (w385:u16)
                    n359 = local read "CAN_1_3"() -> (w384:u16)
                    n360 = local read "CAN_1_4"() -> (w383:u16)
                    n361 = call "CanRevOne.vi"("CANPort"=w387, "data_4"=w383, "data_3"=w384, "data_2"=w385, "data_1"=w386) -> ("接收数据"=w380:u16[], "成功？"=w382:bool)  [unwired: 5 in]
                    n362 = Index Array(array=w380, index #1=0 ("索引"), index #2=1 ("索引"), index #3=2 ("索引"), index #4=3 ("索引")) -> (element #1=w374:u16, element #2=w373:u16, element #3=w372:u16, element #4=w371:u16)
                    n363 = case shown="假" w382 {
                      tunnel: [cluster{u32, u32}[] [{16711680, 16711680}] cluster{u32, u32}[] [{6618880, 6618880}]] -> w375
                      tunnel: [FALSE TRUE] -> w381
                      frame False {
                      }
                      frame True {
                      }
                    }
                    n364 = local write "CAN_R_1_1"(w374) -> ()
                    n365 = local write "CAN_R_1_2"(w373) -> ()
                    n366 = local write "CAN_R_1_3"(w372) -> ()
                    n367 = local write "CAN_R_1_4"(w371) -> ()
                  }
                }
                n368 = property on="light_1" class="Bool (严格)"("Colors [4]"=w366) -> ()  [unwired: 2 in, 2 out]
              }
            }
            n369 = local write "同步_2"(w273) -> ()
            n370 = case shown="假" w274 {
              tunnel: ["CAN通讯故障" "CAN通讯正常"] -> w276
              frame False {
              }
              frame True {
              }
            }
            n371 = Format Into String(format string="第%d路", w273) -> (resulting string=w277:string)  [unwired: 2 in, 1 out]
            n372 = local read "测试结论"() -> (w278:string)
            n373 = Concatenate Strings(w278, w277, w276, "\r") -> (w272:string)
            n374 = local write "测试结论"(w272) -> ()
          }
        }
        n375 = local read "结束?"() -> (w271:bool)
      }
      n376 = Release Notifier(notifier=w258, error in (no error)=w257) -> ()  [unwired: 1 in, 3 out]
    }
    frame Enabled {
    }
  }
